vi "SetLocalPose.vi"(3 "PresenceVector":u16=2 format="%x", 4 "LocalPose":T1, 5 "Destination":T3={"Subsystem Id"=90, "Node Id"=1, "Component Id"=1}, 6 "Source":T3={"Subsystem Id"=3, "Node Id"=1, "Component Id"=1}) -> (1 "Encoded JAUS Message":string)   [LabVIEW 2009]
uses:
  Support Files/Address.ctl
  Support Files/LocalPose.ctl
  Support Files/TimeRec.ctl
panel:
  in  "Send current system time":bool
  in  "Command Code":string="\u0004\u0003"
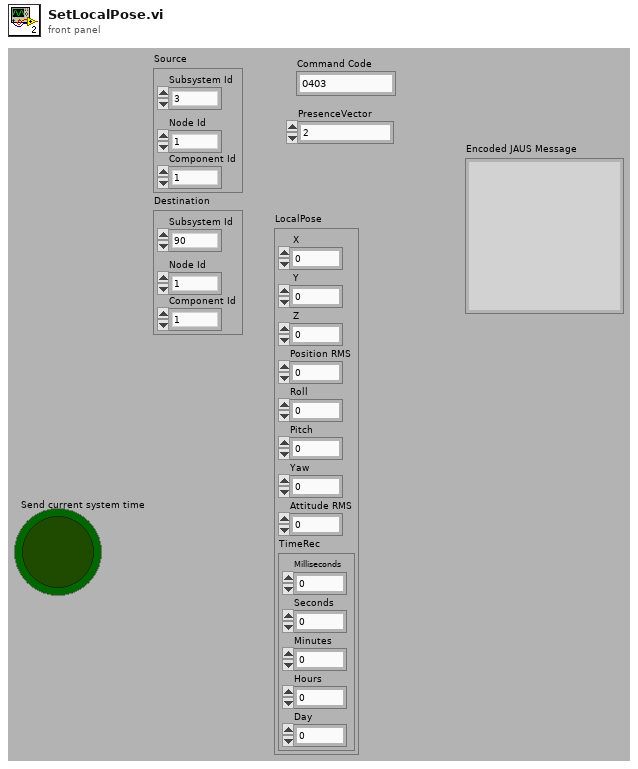
[diagram p1: front panel]
types:
  T1 = typedef "LocalPose.ctl" = cluster{" X":dbl, " Y":dbl, " Z":dbl, "Position RMS":dbl, "Roll":dbl, "Pitch":dbl, "Yaw":dbl, "Attitude RMS":dbl, "TimeRec":T2}
  T2 = typedef "TimeRec.ctl" = cluster{"Milliseconds":u32, "Seconds":u32, "Minutes":u32, "Hours":u32, "Day":u32}
  T3 = typedef "Address.ctl" = cluster{"Subsystem Id":u16, "Node Id":u8, "Component Id":u8}
  T4 = cluster{"unsigned byte array[0]":u8, "unsigned byte array[1]":u8}
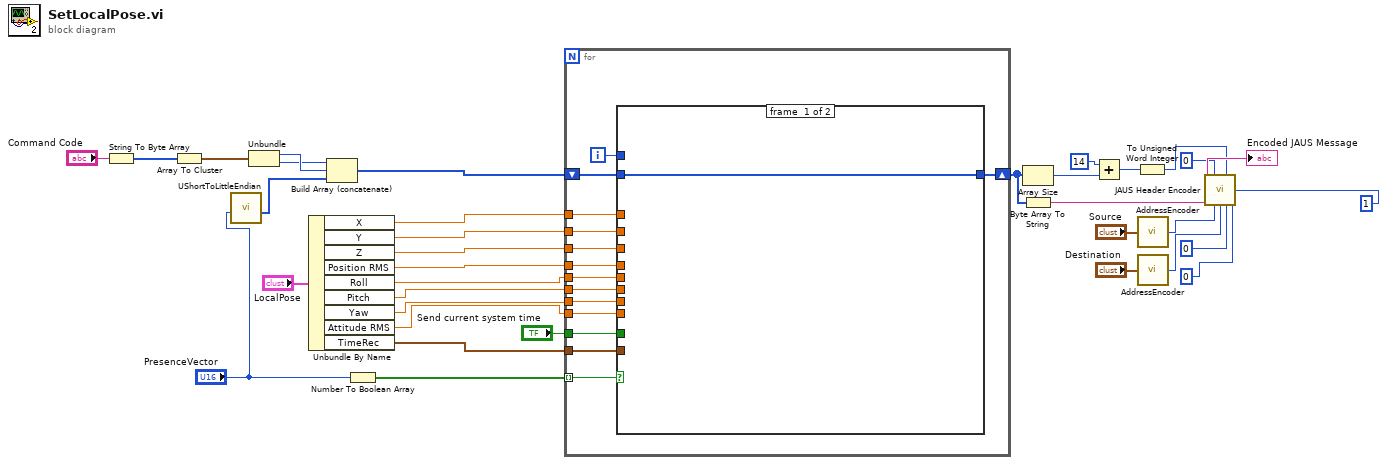
[diagram p0: block diagram]
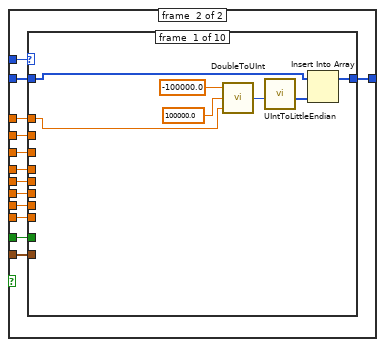
[diagram p2: hidden frame]
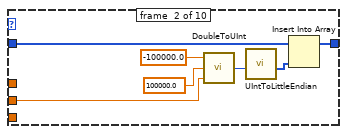
[diagram p3: hidden frame]
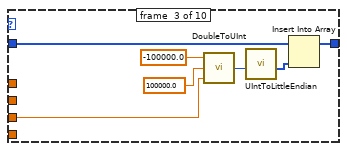
[diagram p4: hidden frame]
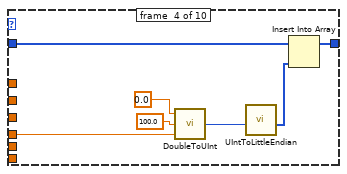
[diagram p5: hidden frame]
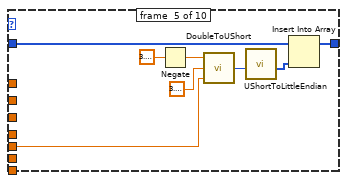
[diagram p6: hidden frame]
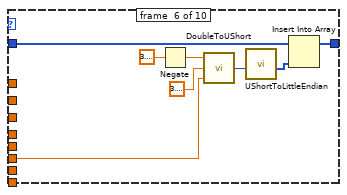
[diagram p7: hidden frame]
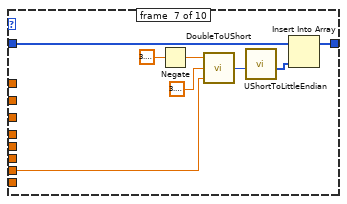
[diagram p8: hidden frame]
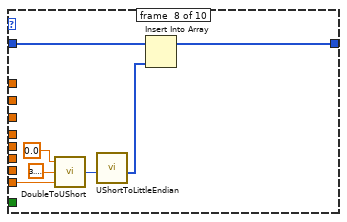
[diagram p9: hidden frame]
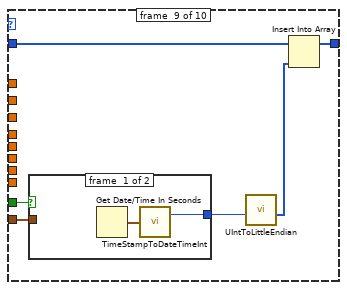
[diagram p10: hidden frame]
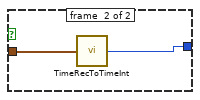
[diagram p11: hidden frame]
diagram:
  n1 = String To Byte Array(string="Command Code") -> (unsigned byte array=w19:u8[])
  n2 = Array To Cluster(array=w19) -> (cluster=w18:T4)
  n3 = call "UShortToLittleEndian.vi"("Number"="PresenceVector") -> ("byte array"=w1:u8[])  [unwired: 10 in]
  n4 = Unbundle(w18) -> ("unsigned byte array[0]"=w17:u8, "unsigned byte array[1]"=w16:u8)
  n5 = Unbundle By Name("LocalPose") -> ("X"=w15:dbl, "Y"=w14:dbl, "Z"=w13:dbl, "Position RMS"=w12:dbl, "Roll"=w11:dbl, "Pitch"=w10:dbl, "Yaw"=w9:dbl, "Attitude RMS"=w8:dbl, "TimeRec"=w7:T2)
  n6 = Build Array (concatenate)(w16, w17, w1) -> (w22:u8[])
  n7 = Number To Boolean Array(number="PresenceVector") -> (Boolean array=w27:bool[])
  n8 = for {
    tunnel: w27 -> [w49] mode=indexing
    tunnel: w15 -> [w47]
    tunnel: w14 -> [w46]
    tunnel: w13 -> [w45]
    tunnel: w12 -> [w44]
    tunnel: w11 -> [w43]
    tunnel: w10 -> [w42]
    tunnel: w9 -> [w41]
    tunnel: w8 -> [w40]
    tunnel: w7 -> [w39]
    tunnel: "Send current system time" -> [w38]
    shift-right: [w36] -> w21
    shift-left: w22 -> [w37]
    i -> [w48]
    n9 = case shown="True" w49 {
      tunnel: w48 -> [_ w63]
      tunnel: w47 -> [_ w62]
      tunnel: w46 -> [_ w61]
      tunnel: w45 -> [_ w60]
      tunnel: w44 -> [_ w59]
      tunnel: w43 -> [_ w58]
      tunnel: w42 -> [_ w57]
      tunnel: w41 -> [_ w56]
      tunnel: w40 -> [_ w55]
      tunnel: w39 -> [_ w54]
      tunnel: w38 -> [_ w53]
      tunnel: w37 -> [w50 w52]
      tunnel: [w50 w51] -> w36
      frame #0 {
      }
      frame #1 {
        n10 = case shown="8" w63 {
          tunnel: w62 -> [w67 _ _ _ _ _ _ _ _ _]
          tunnel: w61 -> [_ w73 _ _ _ _ _ _ _ _]
          tunnel: w60 -> [_ _ w80 _ _ _ _ _ _ _]
          tunnel: w59 -> [_ _ _ w87 _ _ _ _ _ _]
          tunnel: w58 -> [_ _ _ _ w94 _ _ _ _ _]
          tunnel: w57 -> [_ _ _ _ _ w102 _ _ _ _]
          tunnel: w56 -> [_ _ _ _ _ _ w110 _ _ _]
          tunnel: w55 -> [_ _ _ _ _ _ _ w118 _ _]
          tunnel: w54 -> [_ _ _ _ _ _ _ _ w128 _]
          tunnel: w53 -> [_ _ _ _ _ _ _ _ w127 _]
          tunnel: w52 -> [w66 w72 w79 w86 w93 w101 w109 w117 w125 w133]
          tunnel: [w65 w71 w78 w85 w92 w100 w108 w116 w123 w133] -> w51
          frame #0 {
            n11 = call "DoubleToUInt.vi"("Value"=w67, "Max"=100000.0, "Min"=-100000.0) -> ("scaled Integer"=w64:u32)
            n12 = call "UIntToLittleEndian.vi"("Number"=w64) -> ("byte array"=w68:u8[])  [unwired: 10 in]
            n13 = Insert Into Array(array=w66, new element=w68) -> (w65:u8[])  [unwired: 1 in]
          }
          frame #1 {
            n14 = call "DoubleToUInt.vi"("Value"=w73, "Max"=100000.0, "Min"=-100000.0) -> ("scaled Integer"=w75:u32)
            n15 = call "UIntToLittleEndian.vi"("Number"=w75) -> ("byte array"=w74:u8[])  [unwired: 10 in]
            n16 = Insert Into Array(array=w72, new element=w74) -> (w71:u8[])  [unwired: 1 in]
          }
          frame #2 {
            n17 = call "DoubleToUInt.vi"("Value"=w80, "Max"=100000.0, "Min"=-100000.0) -> ("scaled Integer"=w82:u32)
            n18 = call "UIntToLittleEndian.vi"("Number"=w82) -> ("byte array"=w81:u8[])  [unwired: 10 in]
            n19 = Insert Into Array(array=w79, new element=w81) -> (w78:u8[])  [unwired: 1 in]
          }
          frame #3 {
            n20 = call "DoubleToUInt.vi"("Value"=w87, "Max"=100.0, "Min"=0.0) -> ("scaled Integer"=w89:u32)
            n21 = call "UIntToLittleEndian.vi"("Number"=w89) -> ("byte array"=w88:u8[])  [unwired: 10 in]
            n22 = Insert Into Array(array=w86, new element=w88) -> (w85:u8[])  [unwired: 1 in]
          }
          frame #4 {
            n23 = Negate(x=3.141592653589793) -> (-x=w95:dbl)
            n24 = call "DoubleToUShort.vi"("Value"=w94, "Max"=3.141592653589793, "Min"=w95) -> ("scaled Integer"=w99:u16)
            n25 = call "UShortToLittleEndian.vi"("Number"=w99) -> ("byte array"=w98:u8[])  [unwired: 10 in]
            n26 = Insert Into Array(array=w93, new element=w98) -> (w92:u8[])  [unwired: 1 in]
          }
          frame #5 {
            n27 = Negate(x=3.141592653589793) -> (-x=w104:dbl)
            n28 = call "DoubleToUShort.vi"("Value"=w102, "Max"=3.141592653589793, "Min"=w104) -> ("scaled Integer"=w107:u16)
            n29 = call "UShortToLittleEndian.vi"("Number"=w107) -> ("byte array"=w106:u8[])  [unwired: 10 in]
            n30 = Insert Into Array(array=w101, new element=w106) -> (w100:u8[])  [unwired: 1 in]
          }
          frame #6 {
            n31 = Negate(x=3.141592653589793) -> (-x=w112:dbl)
            n32 = call "DoubleToUShort.vi"("Value"=w110, "Max"=3.141592653589793, "Min"=w112) -> ("scaled Integer"=w115:u16)
            n33 = call "UShortToLittleEndian.vi"("Number"=w115) -> ("byte array"=w114:u8[])  [unwired: 10 in]
            n34 = Insert Into Array(array=w109, new element=w114) -> (w108:u8[])  [unwired: 1 in]
          }
          frame #7 {
            n35 = call "DoubleToUShort.vi"("Value"=w118, "Max"=3.141592653589793, "Min"=0.0) -> ("scaled Integer"=w122:u16)
            n36 = call "UShortToLittleEndian.vi"("Number"=w122) -> ("byte array"=w121:u8[])  [unwired: 10 in]
            n37 = Insert Into Array(array=w117, new element=w121) -> (w116:u8[])  [unwired: 1 in]
          }
          frame #8 {
            n38 = case shown="True" w127 {
              tunnel: w128 -> [_ w132]
              tunnel: [w129 w131] -> w124
              frame #0 {
                n39 = Get Date/Time In Seconds() -> (seconds since 1Jan1904=w130:timestamp)
                n40 = call "TimeStampToDateTimeInt.vi"("Time Stamp"=w130) -> ("timeInt"=w129:u32)  [unwired: 1 out]
              }
              frame #1 {
                n41 = call "TimeRecToTimeInt.vi"("TimeRec"=w132) -> ("timeInt"=w131:u32)
              }
            }
            n42 = call "UIntToLittleEndian.vi"("Number"=w124) -> ("byte array"=w126:u8[])  [unwired: 10 in]
            n43 = Insert Into Array(array=w125, new element=w126) -> (w123:u8[])  [unwired: 1 in]
          }
          frame #9 {
          }
        }
      }
    }
  }
  n44 = Array Size(array=w21) -> (size(s)=w5:i32)
  n45 = Byte Array To String(unsigned byte array=w21) -> (string=w26:string)
  n46 = Add(x=14, y=w5) -> (x+y=w4:i32)
  n47 = To Unsigned Word Integer(number=w4) -> (unsigned 16bit integer=w23:u16)
  n48 = call "AddressEncoder.vi"("Address Cluster"="Source") -> ("Address"=w34:u32)
  n49 = call "AddressEncoder.vi"("Address Cluster"="Destination") -> ("Address"=w33:u32)
  n50 = call "JAUS Header Encoder.vi"("Message Type (0-5)"=u8 0, "Data Size (8-23)"=w23, "Priority(40-41)"=u8 1, "Payload"=w26, "Source ID (80-95)"=w34, "Destination ID (48-79)"=w33, "Data Flags (46-47)"=u8 0, "Ack/Nak (44-45)"=u8 0) -> ("Encoded JAUS Message"=→"Encoded JAUS Message":string)  [unwired: 7 in]
